vi "General Use dB.vi"(8 "error in (no error)":errorcluster, 11 "Query":string="SELECT * FROM data") -> (0 "error out":errorcluster, 1 "Return Data":variant[][](array[variant]))   [LabVIEW 2020]
uses:
  typedefs/mysql_authentication.ctl
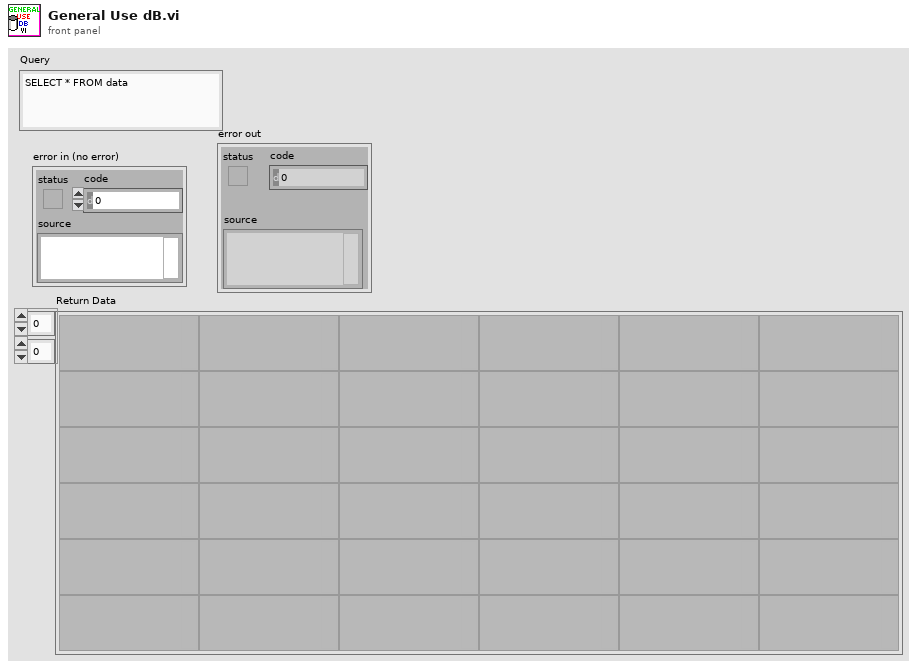
[diagram p1: front panel]
types:
  T1 = typedef "mysql_authentication.ctl" = cluster{"User":string, "Password":string, "Database":string}
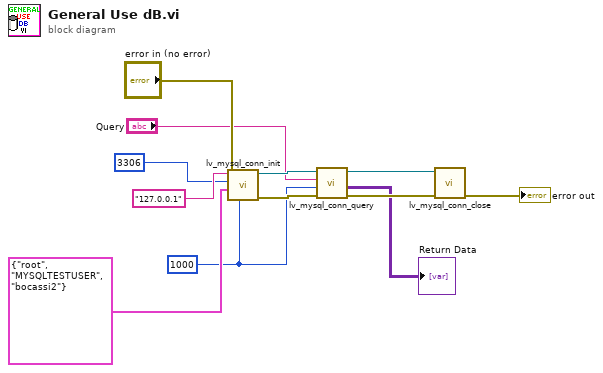
[diagram p0: block diagram]
diagram:
  w6 = 1000 ("timeout ms (60000)")
  n1 = call "lv_mysql_conn_init.vi"("timeout ms (5000)"=w6, "error in (no error)"="error in (no error)", "Authentication"=T1 {"User"="root", "Password"="MYSQLTESTUSER", "Database"="bocassi2"}, "Port"=u16 3306, "IP Address"="127.0.0.1") -> ("error out"=w9:errorcluster, "connection ID out"=w8:refnum<k5>)  [unwired: 5 in]
  n2 = call "lv_mysql_conn_query.vi"("error in (no error)"=w9, "timeout ms (5000)"=w6, "Query"="Query", "connection ID"=w8) -> ("error out"=w4:errorcluster, "Return Data"=→"Return Data":variant[][], "connection ID out"=w7:refnum<k5>)  [unwired: 4 in, 1 out]
  n3 = call "lv_mysql_conn_close.vi"("error in (no error)"=w4, "connection ID"=w7) -> ("error out"=→"error out":errorcluster)  [unwired: 9 in]
